vi "SUB_COM1_CLOSE.vi"(3 "VISA resource name":refnum<visa-resource-name>) -> ()   [LabVIEW 2011]
uses:
  <vilib>/Instr/_visa.llb/VISA Flush IO Buffer Mask.ctl
panel:
  out "error out":errorcluster
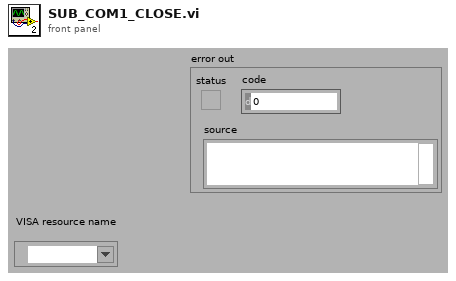
[diagram p1: front panel]
types:
  T1 = typedef "VISA Flush IO Buffer Mask.ctl" = u16
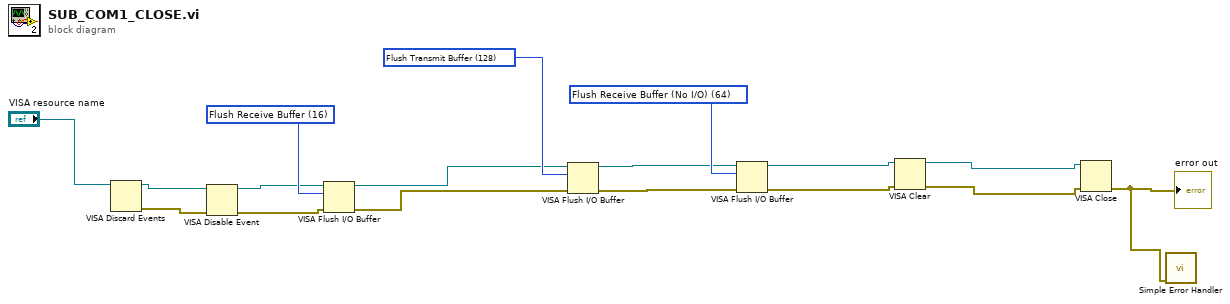
[diagram p0: block diagram]
diagram:
  w9 = T1 16 items=["Flush Receive Buffer"=16, "Write Transmit Buffer to Device"=32, "Flush Receive Buffer (No I/O)"=64, "Flush Transmit Buffer"=128] ("Mask")
  w14 = T1 64 items=["Flush Receive Buffer"=16, "Write Transmit Buffer to Device"=32, "Flush Receive Buffer (No I/O)"=64, "Flush Transmit Buffer"=128] ("Mask")
  w17 = T1 128 items=["Flush Receive Buffer"=16, "Write Transmit Buffer to Device"=32, "Flush Receive Buffer (No I/O)"=64, "Flush Transmit Buffer"=128] ("Mask")
  n1 = VISA Discard Events(11:"VISA resource name") -> (0:w2:errorcluster, 3:w5:refnum<visa-resource-name>)  [unwired: 3 in]
  n2 = VISA Disable Event(8:w2, 11:w5) -> (0:w3:errorcluster, 3:w4:refnum<visa-resource-name>)  [unwired: 2 in]
  n3 = VISA Flush I/O Buffer(VISA resource name=w4, mask (16)=w9, error in (no error)=w3) -> (VISA resource name out=w8:refnum<visa-resource-name>, error out=w7:errorcluster)
  n4 = VISA Flush I/O Buffer(VISA resource name=w8, mask (16)=w17, error in (no error)=w7) -> (VISA resource name out=w13:refnum<visa-resource-name>, error out=w12:errorcluster)
  n5 = VISA Flush I/O Buffer(VISA resource name=w13, mask (16)=w14, error in (no error)=w12) -> (VISA resource name out=w11:refnum<visa-resource-name>, error out=w10:errorcluster)
  n6 = VISA Clear(VISA resource name=w11, error in (no error)=w10) -> (VISA resource name out=w16:refnum<visa-resource-name>, error out=w15:errorcluster)
  n7 = VISA Close(VISA resource name=w16, error in (no error)=w15) -> (error out=w1:errorcluster)
  "error out" <- w1
  n8 = call <vilib>:"Simple Error Handler.vi"("error in (no error)"=w1) -> ()  [unwired: 1 in, 8 out]
